vi "LabVIEW to TOML.vi"(8 "error in (no error)":errorcluster, 11 "LV Value":variant) -> (0 "error out":errorcluster, 3 "TOML Value":T1)   [LabVIEW 2019, in "BlueTOMLSerializer.lvlib"]
uses:
  BlueTOMLSerializer.lvlib
  TOML Value.ctl
  Value.ctl
  Value Type.ctl
  Key-Value Pair.ctl
  <vilib>/Utility/Data Type/NI_Data Type.lvlib
  <vilib>/JDP Science/JDP Science Common Utilities/JDP Utility.lvlib
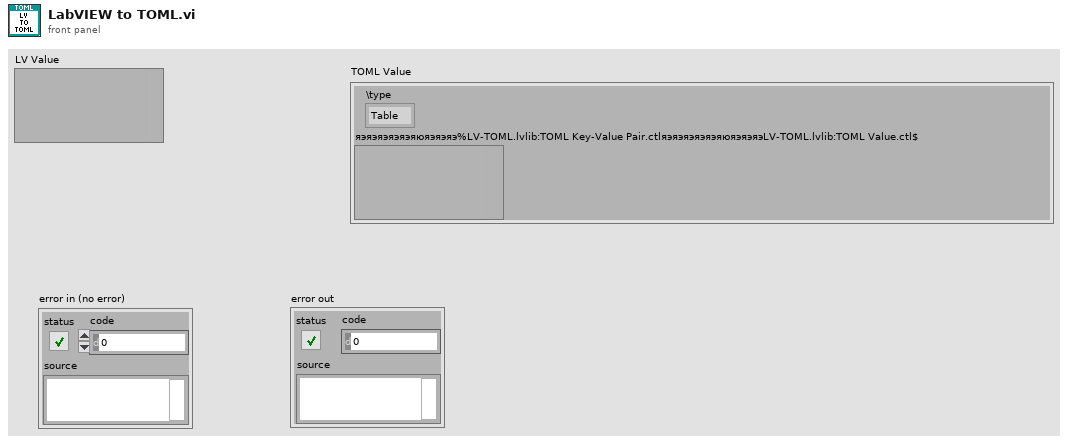
[diagram p1: front panel]
types:
  T1 = typedef "BlueTOMLSerializer.lvlib/TOML Value.ctl" = cluster{"\\type":enum16{"Table", "Array", "String", "Integer", "Float", "Boolean", "Offset Date-Time", "Local Date-Time", "Local Date", "Local Time"}, "яэяэяэяэяэяюяэяэяэ%LV-TOML.lvlib:TOML Key-Value Pair.ctlяэяэяэяэяэяюяэяэяэLV-TOML.lvlib:TOML Value.ctl$":variant}
  T2 = typedef "BlueTOMLSerializer.lvlib/Value.ctl" = cluster{"Type":T3, "Value":variant}
  T3 = typedef "BlueTOMLSerializer.lvlib/Value Type.ctl" = enum16{"Table", "Array", "String", "Integer", "Float", "Boolean", "Offset Date-Time", "Local Date-Time", "Local Date", "Local Time"}
  T4 = typedef "BlueTOMLSerializer.lvlib/Key-Value Pair.ctl" = cluster{"Key":string, "Value":T2}
  T5 = typedef "NI_Data Type.lvlib/Data Type.ctl" = enum8{"Invalid Type", "Void", "I8", "I16", "I32", "I64", "U8", "U16", "U32", "U64", "Single Float", "Double Float", "Extended Float", "Single Complex", "Double Complex", "Extended Complex", "Enum U8", "Enum U16", "Enum U32", "Enum U64", "Single Float With Unit", "Double Float With Unit", "Extended Float With Unit", "Single Complex with Unit", "Double Complex with Unit", "Extended Complex with Unit", "Boolean", "String", "Path", "Picture", "Tag", "Array", "Cluster", "Variant", "LV Variant", "Waveform", "Timestamp", "Digital Waveform", "Digital Data", "ExpressData", "Refnum", "External Data", "VI", "Poly VI", "LabVIEW Class Instance", "Fixed Point", "Set Collection", "Map Collection"}
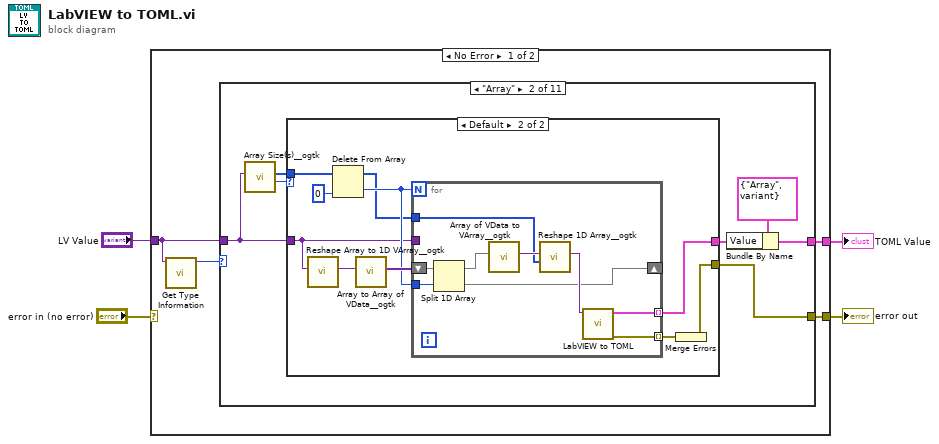
[diagram p0: block diagram]
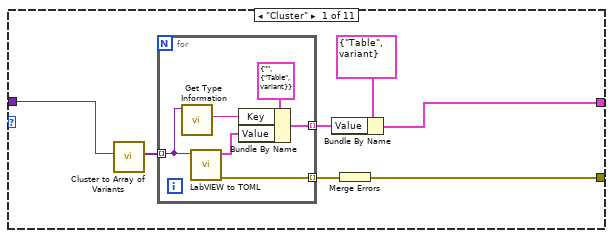
[diagram p2: hidden frame]
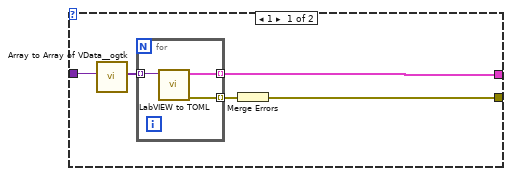
[diagram p3: hidden frame]
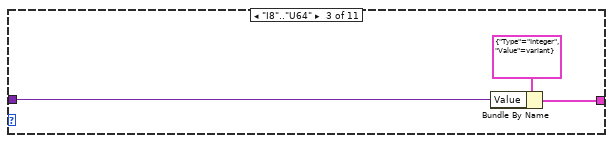
[diagram p4: hidden frame]
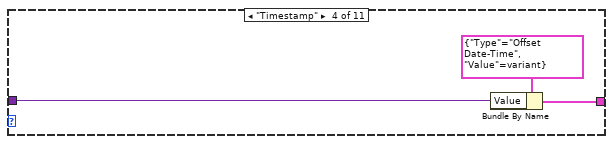
[diagram p5: hidden frame]
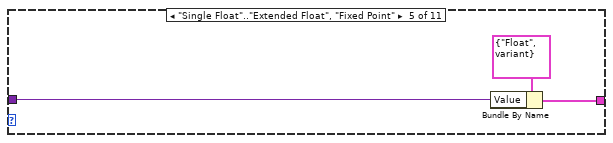
[diagram p6: hidden frame]
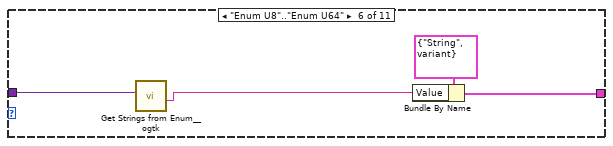
[diagram p7: hidden frame]
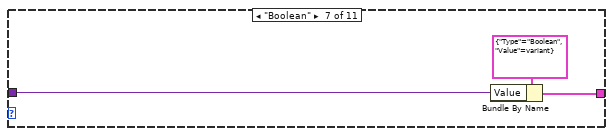
[diagram p8: hidden frame]
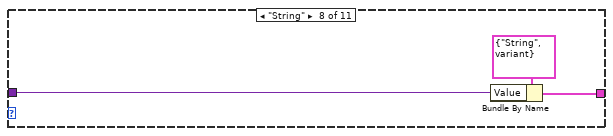
[diagram p9: hidden frame]
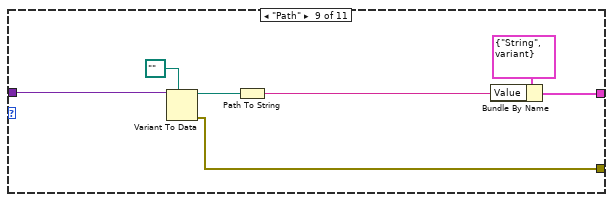
[diagram p10: hidden frame]
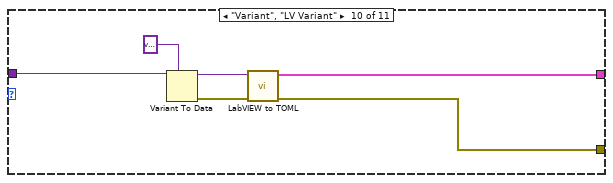
[diagram p11: hidden frame]
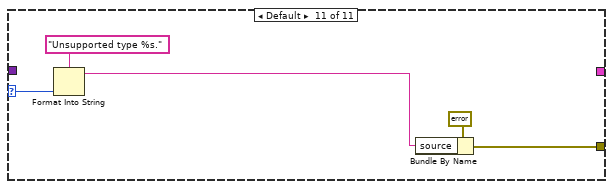
[diagram p12: hidden frame]
diagram:
  n1 = case shown="No Error" "error in (no error)" {
    selector: "error in (no error)" -> [_ w93]
    tunnel: "LV Value" -> [w6 _]
    tunnel: [w7 _] -> w3
    tunnel: [w5 w93] -> w1
    frame No Error {
      n2 = call <vilib>:"Get Type Information.vi"("variant"=w6) -> ("type"=w8:T5)  [unwired: 6 in, 4 out]
      n3 = case shown="\"Array\"" w8 {
        selector: w8 -> [_ _ _ _ _ _ _ _ _ _ w92]
        tunnel: w6 -> [w10 w28 w56 w59 w62 w68 w69 w72 w78 w87 _]
        tunnel: [w13 w24 w58 w61 w64 w65 w71 w74 w81 w83 _] -> w7
        tunnel: [w11 w22 _ _ _ _ _ _ w76 w82 w89] -> w5
        frame "Cluster" {
          n4 = call <vilib>:"Cluster to Array of Variants.vi"("Cluster"=w10) -> ("Array of Cluster Elements"=w9:variant[])  [unwired: 10 in]
          n5 = for {
            tunnel: w9 -> [w21] mode=indexing
            tunnel: [w17] -> w15 mode=indexing
            tunnel: [w16] -> w12 mode=indexing
            n6 = call <vilib>:"Get Type Information.vi"("variant"=w21) -> ("name"=w19:string)  [unwired: 6 in, 4 out]
            n7 = call "LabVIEW to TOML.vi"("LV Value"=w21) -> ("error out"=w16:errorcluster, "TOML Value"=w18:T1)  [unwired: 9 in]
            n8 = Bundle By Name(cluster=T4 {"Key"="", "Value"={"Type"=enum."Table", "Value"=variant}} ("Key-Value Pair"), "Key"=w19, "Value"=w18) -> (w17:T4)
          }
          n9 = Bundle By Name(cluster=T2 {"Type"=enum."Table", "Value"=variant} ("Value"), "Value"=w15) -> (w13:T2)
          n10 = Merge Errors(w12) -> (w11:errorcluster)
        }
        frame "Array" {
          n11 = call <userlib>:"Array Size(s)__ogtk.vi"("Array"=w28) -> ("N dims"=w26:u32, "Size(s)"=w27:u32[])  [unwired: 8 in, 1 out]
          n12 = case shown="Default" w26 {
            tunnel: w28 -> [w33 w39]
            tunnel: w27 -> [_ w43]
            tunnel: [w31 w40] -> w25
            tunnel: [w29 w37] -> w22
            frame 1 {
              n13 = call <userlib>:"Array to Array of VData__ogtk.vi"("MultiD Array"=w33) -> ("1D Array of Variants"=w32:variant[])  [unwired: 9 in, 1 out]
              n14 = for {
                tunnel: w32 -> [w36] mode=indexing
                tunnel: [w35] -> w31 mode=indexing
                tunnel: [w34] -> w30 mode=indexing
                n15 = call "LabVIEW to TOML.vi"("LV Value"=w36) -> ("error out"=w34:errorcluster, "TOML Value"=w35:T1)  [unwired: 9 in]
              }
              n16 = Merge Errors(w30) -> (w29:errorcluster)
            }
            frame Default {
              n17 = call <userlib>:"Reshape Array to 1D VArray__ogtk.vi"("MultiD Array"=w39) -> ("1D VArray"=w46:variant)  [unwired: 8 in, 2 out]
              n18 = Delete From Array(array=w43, index=0) -> (deleted portion=w42:u32, array with subset deleted=w41:u32[])  [unwired: 1 in]
              n19 = call <userlib>:"Array to Array of VData__ogtk.vi"("MultiD Array"=w46) -> ("1D Array of Variants"=w45:variant[])  [unwired: 9 in, 1 out]
              n20 = for {
                N: w42 -> [_]
                tunnel: w39 -> [_]
                shift-right: [w48] -> _
                shift-left: w45 -> [w55]
                tunnel: w42 -> [w54]
                tunnel: w41 -> [w52]
                tunnel: [w50] -> w40 mode=indexing
                tunnel: [w47] -> w38 mode=indexing
                n21 = Split 1D Array(array=w55, index=w54) -> (first subarray=w49:variant[], second subarray=w48:variant[])
                n22 = call <userlib>:"Array of VData to VArray__ogtk.vi"("1D Array of VData"=w49) -> ("VArray"=w53:variant)  [unwired: 9 in, 1 out]
                n23 = call <userlib>:"Reshape 1D Array__ogtk.vi"("Size(s)"=w52, "1D Array"=w53) -> ("Reshaped VArray"=w51:variant)  [unwired: 8 in, 1 out]
                n24 = call "LabVIEW to TOML.vi"("LV Value"=w51) -> ("error out"=w47:errorcluster, "TOML Value"=w50:T1)  [unwired: 9 in]
              }
              n25 = Merge Errors(w38) -> (w37:errorcluster)
            }
          }
          n26 = Bundle By Name(cluster=T2 {"Type"=enum."Array", "Value"=variant} ("Value"), "Value"=w25) -> (w24:T2)
        }
        frame "I8".."U64" {
          n27 = Bundle By Name(cluster=T2 {"Type"=enum."Integer", "Value"=variant} ("Value"), "Value"=w56) -> (w58:T2)
        }
        frame "Timestamp" {
          n28 = Bundle By Name(cluster=T2 {"Type"=enum."Offset Date-Time", "Value"=variant} ("Value"), "Value"=w59) -> (w61:T2)
        }
        frame "Single Float".."Extended Float", "Fixed Point" {
          n29 = Bundle By Name(cluster=T2 {"Type"=enum."Float", "Value"=variant} ("Value"), "Value"=w62) -> (w64:T2)
        }
        frame "Enum U8".."Enum U64" {
          n30 = call <userlib>:"Get Strings from Enum__ogtk.vi"("Enum"=w68) -> ("String Value"=w66:string)  [unwired: 7 in, 3 out]
          n31 = Bundle By Name(cluster=T2 {"Type"=enum."String", "Value"=variant} ("Value"), "Value"=w66) -> (w65:T2)
        }
        frame "Boolean" {
          n32 = Bundle By Name(cluster=T2 {"Type"=enum."Boolean", "Value"=variant} ("Value"), "Value"=w69) -> (w71:T2)
        }
        frame "String" {
          n33 = Bundle By Name(cluster=T2 {"Type"=enum."String", "Value"=variant} ("Value"), "Value"=w72) -> (w74:T2)
        }
        frame "Path" {
          n34 = Variant To Data(type=path "", Variant=w78) -> (data=w77:path, error out=w76:errorcluster)  [unwired: 1 in]
          n35 = Path To String(path=w77) -> (string=w75:string)
          n36 = Bundle By Name(cluster=T2 {"Type"=enum."String", "Value"=variant} ("Value"), "Value"=w75) -> (w81:T2)
        }
        frame "Variant", "LV Variant" {
          n37 = Variant To Data(type=variant, Variant=w87) -> (data=w84:variant, error out=w85:errorcluster)  [unwired: 1 in]
          n38 = call "LabVIEW to TOML.vi"("error in (no error)"=w85, "LV Value"=w84) -> ("error out"=w82:errorcluster, "TOML Value"=w83:T1)  [unwired: 8 in]
        }
        frame Default {
          n39 = Format Into String(format string="Unsupported type %s.", w92) -> (resulting string=w88:string)  [unwired: 2 in, 1 out]
          n40 = Bundle By Name(cluster=errorcluster {"status"=TRUE, "code"=5001, "source"=""} ("error IO"), "source"=w88) -> (w89:errorcluster)
        }
      }
    }
    frame Error {
    }
  }
  "error out" <- w1
  "TOML Value" <- w3
